vi "Stop_Watch.vi"(0 "Control_Cluster":T2, 5 "Stop":bool) -> (4 "Time_Display":T1 {"ms" format="%#.2g"})   [LabVIEW 2023]
doc: "This VI is a digital stop watch, which does the Same operations of normal Stop watches."
uses:
  Controls/Control_Cluster.ctl
  Controls/Time_Display.ctl
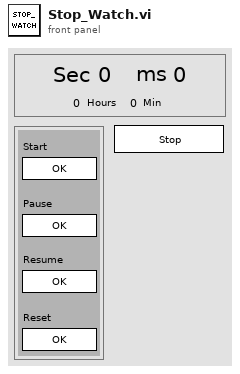
[diagram p1: front panel]
types:
  T1 = typedef "Time_Display.ctl" = cluster{"Hours":i32, "Min":i32, "Sec":i32, "ms":i32}
  T2 = typedef "Control_Cluster.ctl" = cluster{"Start":bool, "Pause":bool, "Resume":bool, "Reset":bool}
  T3 = typedef "LVDateTimeRec.ctl" = cluster{"fractional second":dbl, "second":i32, "minute":i32, "hour":i32, "day of month":i32, "month":i32, "year":i32, "day of week":i32, "day of year":i32, "DST":i32}
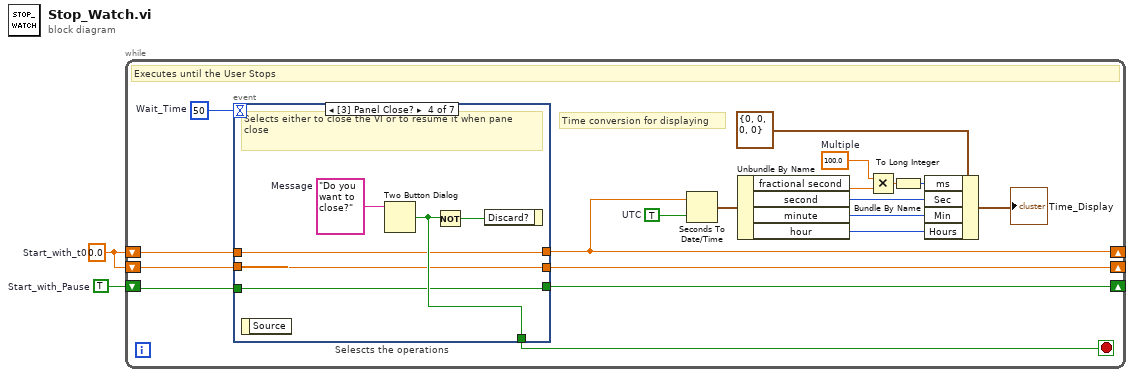
[diagram p0: block diagram]
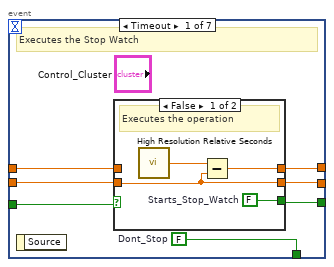
[diagram p2: hidden frame]
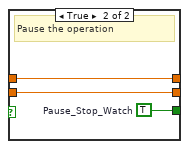
[diagram p3: hidden frame]
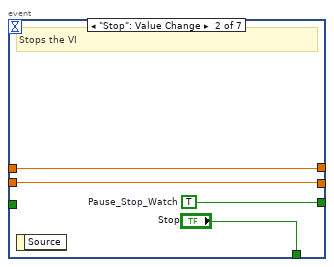
[diagram p4: hidden frame]
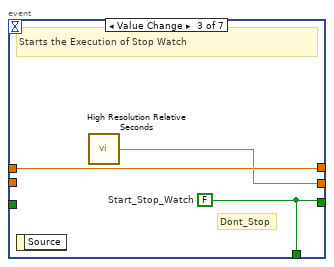
[diagram p5: hidden frame]
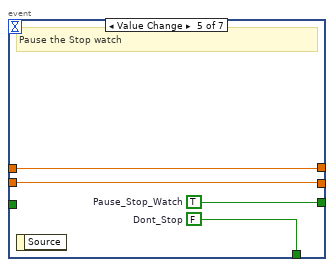
[diagram p6: hidden frame]
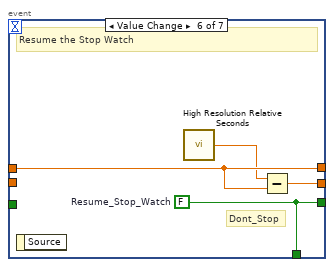
[diagram p7: hidden frame]
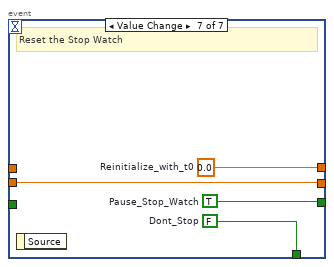
[diagram p8: hidden frame]
diagram:
  w1 = 0.0  # Start_with_t0
  w2 = TRUE  # Start_with_Pause
  n1 = while {
    shift-right: [w19] -> _
    shift-left: w2 -> [w20]
    shift-right: [w17] -> _
    shift-left: w1 -> [w15]
    shift-right: [w8] -> _
    shift-left: w1 -> [w16]
    stop <- w18 stop-if-true
    w4 = 100.0  # Multiple
    w9 = TRUE  # UTC
    w21 = 50  # Wait_Time
    # "Time conversion for displaying"
    # "Executes until the User Stops"
    n2 = event "Selescts the operations" shown="[3] Panel Close?" {
      selector: _ -> [_ _ _ _ _ _ _]
      dyn-events: _ -> [_ _ _ _ _ _ _]
      timeout: w21 -> [_ _ _ _ _ _ _]
      tunnel: w20 -> [w28 _ _ w43 _ _ _]
      tunnel: [w27 w36 w40 w43 w50 w53 w60] -> w19
      tunnel: [w22 "Stop" w40 w46 w49 w53 w57] -> w18
      tunnel: w15 -> [w26 w38 _ w44 w51 _ w59]
      tunnel: [w25 w38 w41 w44 w51 w56 w59] -> w17
      tunnel: [w23 w37 w42 w45 w52 w55 w58] -> w8
      tunnel: w16 -> [w24 w37 w42 w45 w52 w55 _]
      event Timeout {
        w22 = FALSE  # Dont_Stop
        # "Executes the Stop Watch"
        n3 = event-data() -> ()  [unwired: 1 in, 1 out]
        n4 = case shown="False" w28 {
          tunnel: [w32 w35] -> w27
          tunnel: w26 -> [w31 w34]
          tunnel: [w31 w34] -> w25
          tunnel: [w30 w33] -> w23
          tunnel: w24 -> [_ w33]
          frame False {
            w32 = FALSE  # Starts_Stop_Watch
            # "Executes the operation"
            n5 = call <vilib>:"High Resolution Relative Seconds.vi"() -> ("relative seconds"=w29:dbl)
            n6 = Subtract(x=w29, y=w31) -> (x-y=w30:dbl)
          }
          frame True {
            w35 = TRUE  # Pause_Stop_Watch
            # "Pause the operation"
          }
        }
      }
      event "Stop": Value Change {
        w36 = TRUE  # Pause_Stop_Watch
        # "Stops the VI"
        n7 = event-data() -> ()  [unwired: 1 in, 1 out]
      }
      event Value Change {
        w40 = FALSE  # Start_Stop_Watch
        # "Dont_Stop"
        # "Starts the Execution of Stop Watch"
        n8 = event-data() -> ()  [unwired: 1 in, 1 out]
        n9 = call <vilib>:"High Resolution Relative Seconds.vi"() -> ("relative seconds"=w41:dbl)
      }
      event Panel Close? {
        w48 = "Do you want to close?"  # Message
        # "Selects either to close the VI or to resume it when pane close"
        n10 = event-data() -> ()  [unwired: 1 in, 1 out]
        n11 = Two Button Dialog(message=w48) -> (T button?=w46:bool)  [unwired: 2 in]
        n12 = Not(x=w46) -> (.not. x?=w47:bool)
        n13 = event-data("Discard?"=w47) -> ()  [unwired: 1 in, 1 out]
      }
      event Value Change {
        w49 = FALSE  # Dont_Stop
        w50 = TRUE  # Pause_Stop_Watch
        # "Pause the Stop watch"
        n14 = event-data() -> ()  [unwired: 1 in, 1 out]
      }
      event Value Change {
        w53 = FALSE  # Resume_Stop_Watch
        # "Dont_Stop"
        # "Resume the Stop Watch"
        n15 = event-data() -> ()  [unwired: 1 in, 1 out]
        n16 = call <vilib>:"High Resolution Relative Seconds.vi"() -> ("relative seconds"=w54:dbl)
        n17 = Subtract(x=w54, y=w55) -> (x-y=w56:dbl)
      }
      event Value Change {
        w57 = FALSE  # Dont_Stop
        w58 = 0.0  # Reinitialize_with_t0
        w60 = TRUE  # Pause_Stop_Watch
        # "Reset the Stop Watch"
        n18 = event-data() -> ()  [unwired: 1 in, 1 out]
      }
    }
    n19 = Seconds To Date/Time(time stamp (now)=w8, to UTC (F)=w9) -> (date time rec=w14:T3)
    n20 = Unbundle By Name(w14) -> ("fractional second"=w6:dbl, "second"=w11:i32, "minute"=w12:i32, "hour"=w13:i32)
    n21 = Multiply(x=w4, y=w6) -> (x*y=w5:dbl)
    n22 = To Long Integer(number=w5) -> (32bit integer=w3:i32)
    n23 = Bundle By Name(cluster=T1 {"Hours"=0, "Min"=0, "Sec"=0, "ms"=0} ("Cluster 3"), "ms"=w3, "Sec"=w11, "Min"=w12, "Hours"=w13) -> (→"Time_Display":T1)
  }
